vi "Init_DM_DUAL_V2.vi"(7 "BM Flat":bool, 8 "BM Flat File":string[](array[string]), 9 "Mirror Modes File":string, 10 "DM Mapping File":string, 11 "Base File Path":path) -> (3 "reference out":refnum<k7>)   [LabVIEW 2014]
uses:
  Controls/Standard Action.ctl
  <vilib>/Utility/file.llb/Read From Spreadsheet File (DBL).vi
  <vilib>/Utility/file.llb/Read From Spreadsheet File (string).vi
panel:
  out "IDs":i32[](array[numeric])
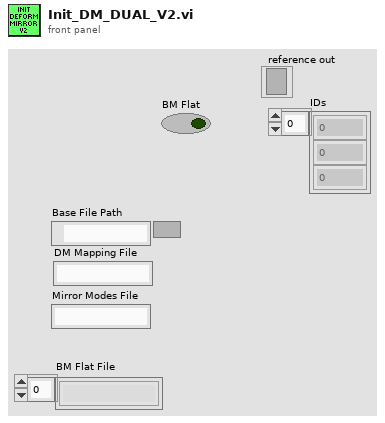
[diagram p1: front panel]
types:
  T1 = typedef "Standard Action.ctl" = enum16{"Read", "Write"}
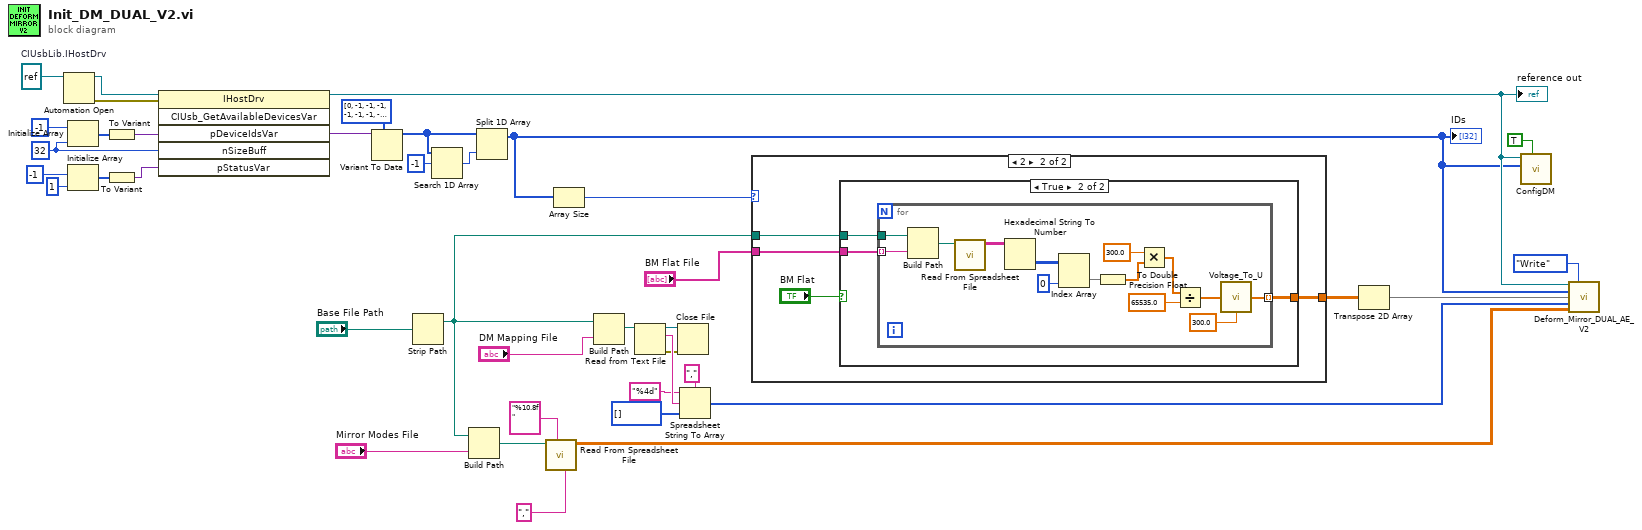
[diagram p0: block diagram]
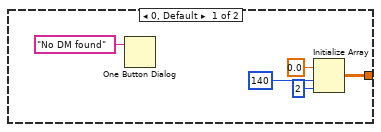
[diagram p2: hidden frame]
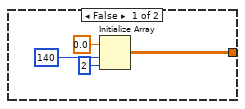
[diagram p3: hidden frame]
diagram:
  w35 = 32 ("dimension size")
  w26 = refnum<k7> refnum  # CIUsbLib.IHostDrv
  n1 = Automation Open(Automation Refnum=w26) -> (Automation Refnum=w31:refnum<k7>, error out=w32:errorcluster)  [unwired: 1 in, 2 out]
  n2 = Initialize Array(-1 ("element"), w35) -> (w28:i32[])
  n3 = Initialize Array(-1 ("element"), 1 ("dimension size")) -> (w27:i32[])
  n4 = To Variant(anything=w28) -> (Variant=w29:variant)
  n5 = To Variant(anything=w27) -> (Variant=w34:variant)
  n6 = invoke class="IHostDrv" method="CIUsb_GetAvailableDevicesVar"(reference=w31, error in=w32, "pDeviceIdsVar"=w29, "nSizeBuff"=w35, "pStatusVar"=w34) -> (reference out=w12:refnum<k7>, "pDeviceIdsVar"=w40:variant)  [unwired: 1 in, 4 out]
  "reference out" <- w12
  n7 = Variant To Data(type=i32[] [0, -1, -1, -1, -1, -1, -1, -1, -1, -1, -1, -1, -1, -1, -1, -1, -1, -1, -1, -1, -1, -1, -1, -1, -1, -1, -1, -1, -1, -1, -1, -1] ("pDeviceIDs"), Variant=w40) -> (data=w38:i32[])  [unwired: 1 in, 1 out]
  n8 = Strip Path(path="Base File Path") -> (stripped path=w16:path)  [unwired: 1 out]
  n9 = Search 1D Array(1D array=w38, element=-1) -> (index of element=w37:i32)  [unwired: 1 in]
  n10 = Build Path(base path=w16, name or relative path="Mirror Modes File") -> (appended path=w17:path)
  n11 = Split 1D Array(array=w38, index=w37) -> (first subarray=w2:i32[])  [unwired: 1 out]
  "IDs" <- w2
  n12 = call-poly <vilib>:"Read From Spreadsheet File.vi"("delimiter (\\t)"="," ("delimiter (\\t)"), "format (%.3f)"="%10.8f", "file path (dialog if empty)"=w17) -> ("all rows"=w7:dbl[][])  [unwired: 2 in, 6 out]
  n13 = Array Size(array=w2) -> (size(s)=w14:i32)
  n14 = Build Path(base path=w16, name or relative path="DM Mapping File") -> (appended path=w19:path)
  n15 = Read from Text File(file (use dialog)=w19) -> (refnum out=w21:refnum<file>, text=w25:string, error out=w20:errorcluster)  [unwired: 1 in, 3 out]
  n16 = Close File(refnum=w21, error in=w20) -> ()  [unwired: 2 out]
  n17 = Spreadsheet String To Array(delimiter (Tab)=",", format string="%4d", spreadsheet string=w25, array type (2D Dbl)=i32[] []) -> (array=w4:i32[])
  n18 = case shown="2" w14 {
    tunnel: w16 -> [_ w49]
    tunnel: "BM Flat File" -> [_ w48]
    tunnel: [w41 w47] -> w3
    frame 0, Default {
      n19 = One Button Dialog(message="No DM found") -> ()  [unwired: 1 in, 1 out]
      n20 = Initialize Array(0.0 ("element"), 140 ("dimension size"), 2 ("dimension size")) -> (w41:dbl[][])
    }
    frame 2 {
      n21 = case shown="True" "BM Flat" {
        tunnel: w49 -> [_ w56]
        tunnel: w48 -> [_ w54]
        tunnel: [w50 w55] -> w47
        frame False {
          n22 = Initialize Array(0.0 ("element"), 140 ("dimension size"), 2 ("dimension size")) -> (w50:dbl[][])
        }
        frame True {
          n23 = for {
            tunnel: w56 -> [w70]
            tunnel: [w57] -> w55 mode=indexing
            tunnel: w54 -> [w60] mode=indexing
            n24 = Build Path(base path=w70, name or relative path=w60) -> (appended path=w69:path)
            n25 = call-poly <vilib>:"Read From Spreadsheet File.vi"("file path (dialog if empty)"=w69) -> ("all rows"=w68:string[][])  [unwired: 3 in, 7 out]
            n26 = Hexadecimal String To Number(string=w68) -> (number=w67:u32[][])  [unwired: 2 in, 1 out]
            n27 = Index Array(array=w67, index (col)=0 ("disabled index (col)")) -> (element=w65:u32[])  [unwired: 1 in]
            n28 = To Double Precision Float(number=w65) -> (double precision float=w61:dbl[])
            n29 = Multiply(x=300.0 ("y"), y=w61) -> (x*y=w64:dbl[])
            n30 = Divide(x=w64, y=65535.0) -> (x/y=w58:dbl[])
            n31 = call "Voltage_To_U.vi"("Voltages In (Volts)"=w58, "Mirror Max Voltage (Volts)"=300.0) -> ("Pixel Value (-1 to 1)"=w57:dbl[])  [unwired: 13 in]
          }
        }
      }
    }
  }
  n32 = Transpose 2D Array(2D array=w3) -> (transposed array=w1:dbl[][])
  n33 = call "ConfigDM.vi"("High Voltage"=TRUE, "Dev IDs"=w2, "Automation Refnum in"=w12) -> ()  [unwired: 7 in, 2 out]
  n34 = call "Deform_Mirror_DUAL_AE_V2.vi"("Refnum In"=w12, "Action"=Standard_Action."Write", "IDs In"=w2, "Flat Files In"=w1, "Multi Map Data In"=w4, "Mode Matrix"=w7) -> ()  [unwired: 5 in, 5 out]
